vi "Check-Create Path.vi"(8 "error in":errorcluster, 11 "Path":path) -> (0 "error out":errorcluster, 3 "Path":path)   [LabVIEW 2011]
doc: "Creates a path if it doesn't exist.\n\n\nVersion 1.0 - 02/13/2013\n\nPhaeron, Inc.\nwww.phaeron.com\ninfo@phaeron.com"
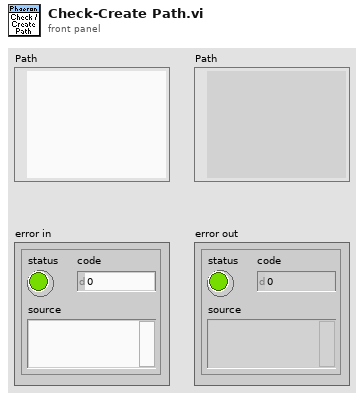
[diagram p1: front panel]
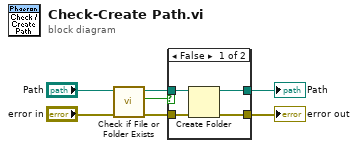
[diagram p0: block diagram]
diagram:
  n1 = call <vilib>:"Check if File or Folder Exists.vi"("error in (no error)"="error in", "path"="Path") -> ("error out"=w6:errorcluster, "file or folder exists?"=w4:bool, "dup path"=w5:path)  [unwired: 7 in]
  n2 = case shown="False" w4 {
    tunnel: [w11 w13] -> w2
    tunnel: [w10 w12] -> w3
    tunnel: w6 -> [w9 w12]
    tunnel: w5 -> [w8 w13]
    frame False {
      n3 = Create Folder(path (use dialog)=w8, error in=w9) -> (created path=w11:path, error out=w10:errorcluster)  [unwired: 1 in, 1 out]
    }
    frame True {
    }
  }
  "Path" <- w2
  "error out" <- w3
